vi "Autonomous Independent.vi"   [LabVIEW 2017]
doc: "This VI is called when autonomous begins, and will automatically be terminated when autonomous ends. You can carry out timed or sensor driven robot movement independently without needing to return to the caller."
uses:
  <vilib>/Rock Robotics/Network Tables/NT Read String.vi
  <vilib>/Rock Robotics/WPI/Utilities/WPI_GetSetVariantRefNum.vi
panel:
  # "Be sure to right-click and choose Data Operations>>Make Current Value default if you want to save the array values with the VI"
types:
  T1 = typedef "WPI_GyroDevRef.ctl" = cluster{"DevStatus":errorcluster, "Analog Channel":T2, "Gain (VoltsPerDegree/Second)":dbl, "Gyro Type":enum16{"Analog", "XRS450"}, "Handle":i32, "SPI Bus":T3, "Device Found":bool, "Sample Rate":dbl, "Calibrate On Open":bool, "Offset":dbl}
  T2 = typedef "FPGA_AIChannel.ctl" = enum8{"AI 0", "AI 1", "AI 2", "AI 3", "AI MXP 0", "AI MXP 1", "AI MXP 2", "AI MXP 3", "Invalid"}
  T3 = typedef "spi_bus.ctl" = enum16{"SPI On-Board, CS0", "SPI On-Board, CS1", "SPI On-Board, CS2", "SPI On-Board, CS3", "SPI MXP", "Invalid"}
  T4 = typedef "WPI_EncoderDevRef.ctl" = cluster{"DevStatus":errorcluster, "EncoderIndex":T5, "CounterIndex":T6, "DistancePerCount":dbl, "Decoding Type":T7}
  T5 = typedef "FPGA_EncoderIdx.ctl" = enum8{"Enc 0", "Enc 1", "Enc 2", "Enc 3", "Enc 4", "Enc 5", "Enc 6", "Enc 7", "Invalid"}
  T6 = typedef "FPGA_CounterCtrSystemIndex.ctl" = enum8{"Ctr 0", "Ctr 1", "Ctr 2", "Ctr 3", "Ctr 4", "Ctr 5", "Ctr 6", "Ctr 7", "Invalid"}
  T7 = typedef "WPI_EncoderType.ctl" = enum16{"1x", "2x", "4x"}
  T8 = typedef "WPI_RobotDriveDevRef.ctl" = cluster{"DevStatus":errorcluster, "Motors[]":T9[], "Square Inputs":bool, "Max Output":dbl}
  T9 = typedef "WPI_MotorControlDeviceRef.ctl" = cluster{"DeviceStatus":errorcluster, "Type":T10, "PWM":cluster{"PWM Channel":T11, "DeadBand":T12}, "CAN":cluster{"Device Number":u8, "SetOutput VI Ref":variant, "GetOutput VI Ref":variant, "Enable VI Ref":variant, "Disable VI Ref":variant, "Data":variant}, "Invert":bool, "DIO PWM":cluster{"PWM \"Enable\" Channel":T11, "DIOChannel":T13, "PWM Rate":dbl}}
  T10 = typedef "WPI_MotorControlType.ctl" = enum16{"PWM", "CAN", "DIO PWM"}
  T11 = typedef "FPGA_DIOPWMChannel.ctl" = enum8{"PWM 0", "PWM 1", "PWM 2", "PWM 3", "PWM 4", "PWM 5", "PWM 6", "PWM 7", "PWM 8", "PWM 9", "PWM MXP 0", "PWM MXP 1", "PWM MXP 2", "PWM MXP 3", "PWM MXP 4", "PWM MXP 5", "PWM MXP 6", "PWM MXP 7", "PWM MXP 8", "PWM MXP 9", "Invalid"}
  T12 = typedef "WPI_PWMDeadband.ctl" = cluster{"Name":string, "maxPositivePwm":i32, "minPositivePwm":i32, "centerPwm":i32, "maxNegativePwm":i32, "minNegativePwm":i32, "angularRange":u16}
  T13 = typedef "FPGA_DIOChannel.ctl" = enum8{"DIO 0", "DIO 1", "DIO 2", "DIO 3", "DIO 4", "DIO 5", "DIO 6", "DIO 7", "DIO 8", "DIO 9", "DIO MXP 0", "DIO MXP 1", "DIO MXP 2", "DIO MXP 3", "DIO MXP 4", "DIO MXP 5", "DIO MXP 6", "DIO MXP 7", "DIO MXP 8", "DIO MXP 9", "DIO MXP 10", "DIO MXP 11", "DIO MXP 12", "DIO MXP 13", "DIO MXP 14", "DIO MXP 15", "SPI Port CS1", "SPI Port CS2", "SPI Port CS3", "SPI Port MISO", "SPI Port MOSI", "Invalid"}
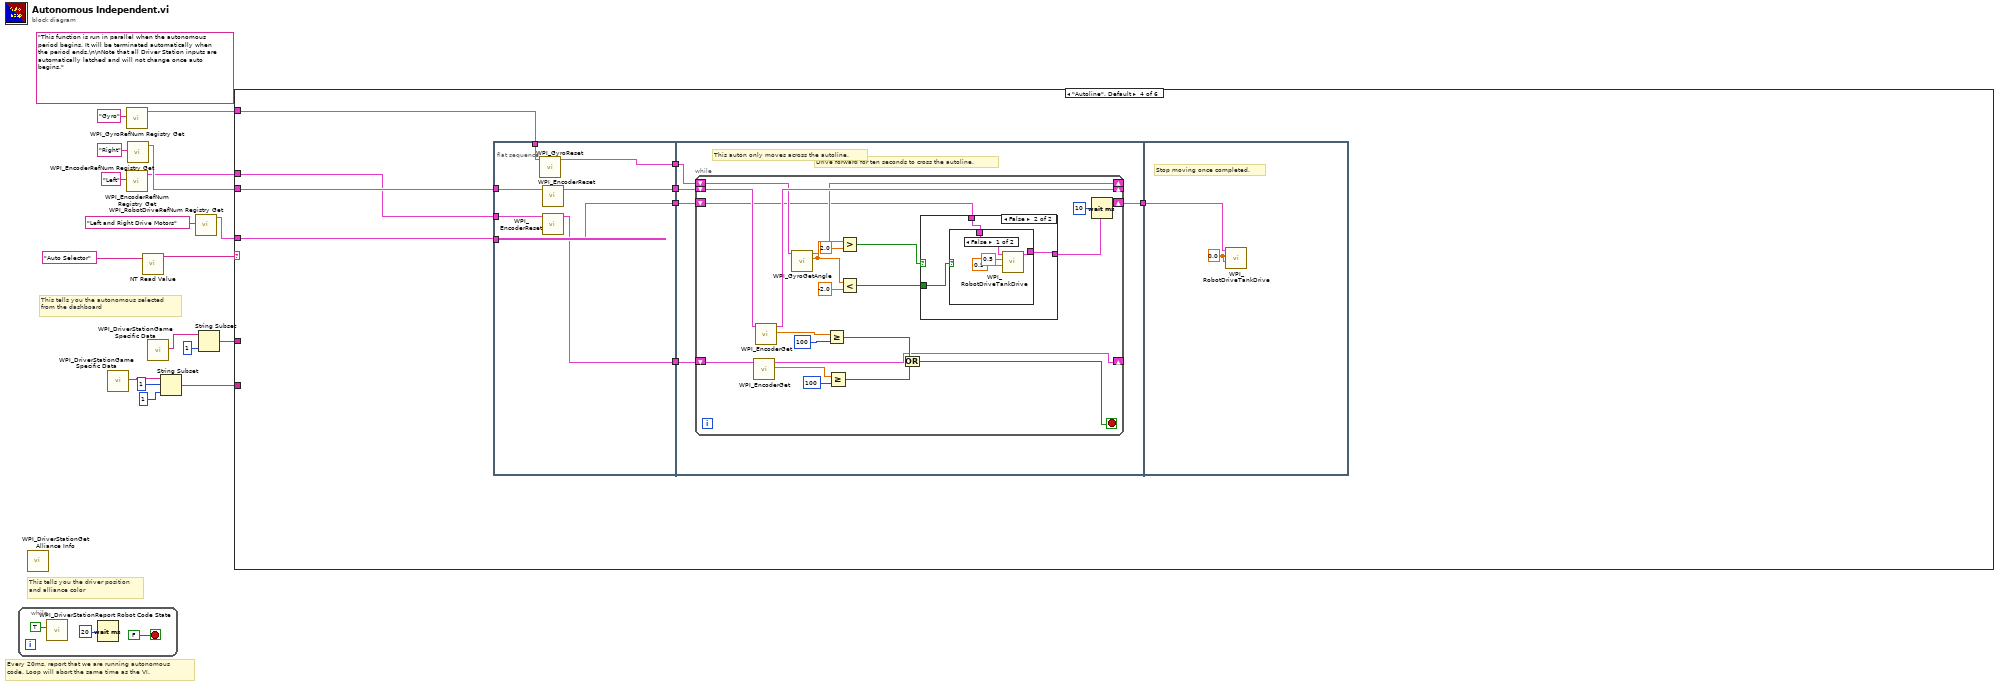
[diagram p0: block diagram]
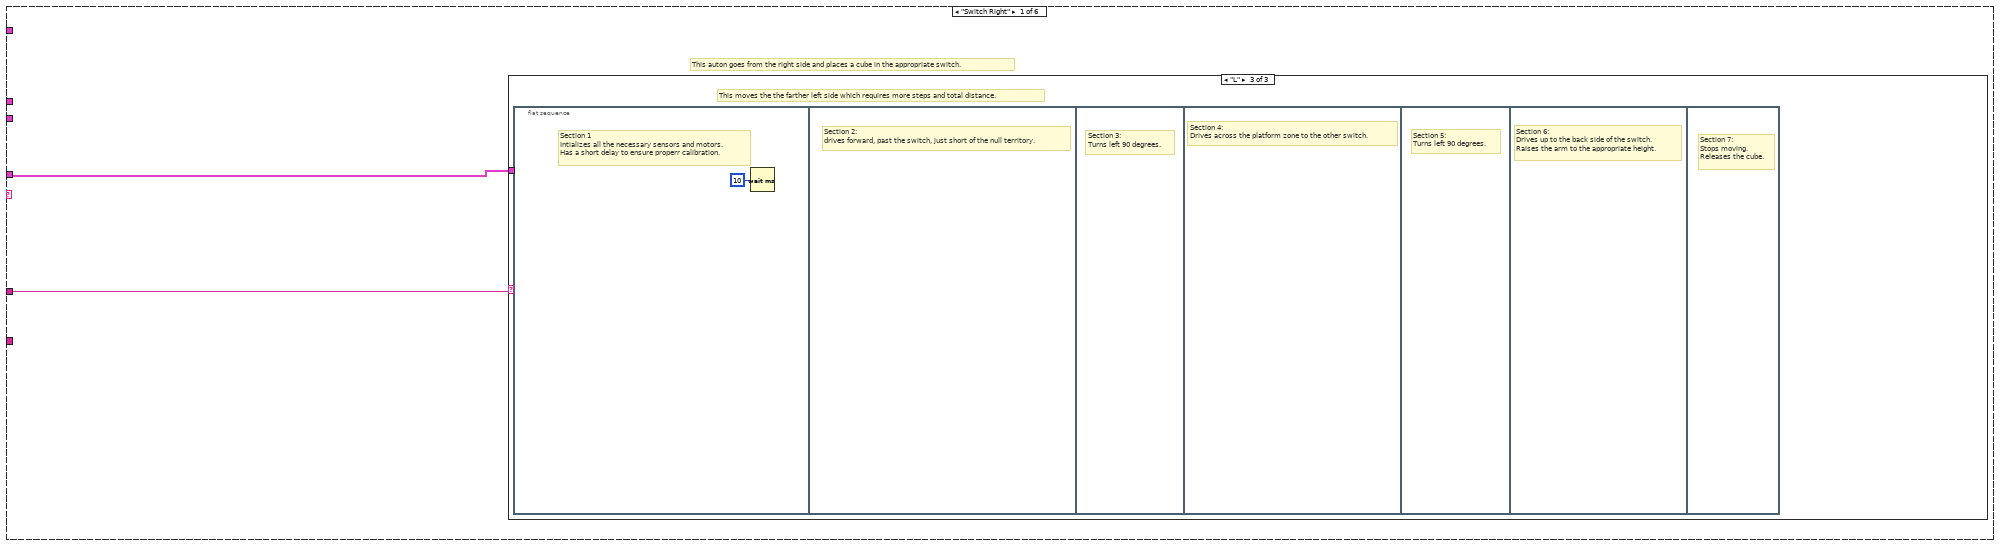
[diagram p2: hidden frame]
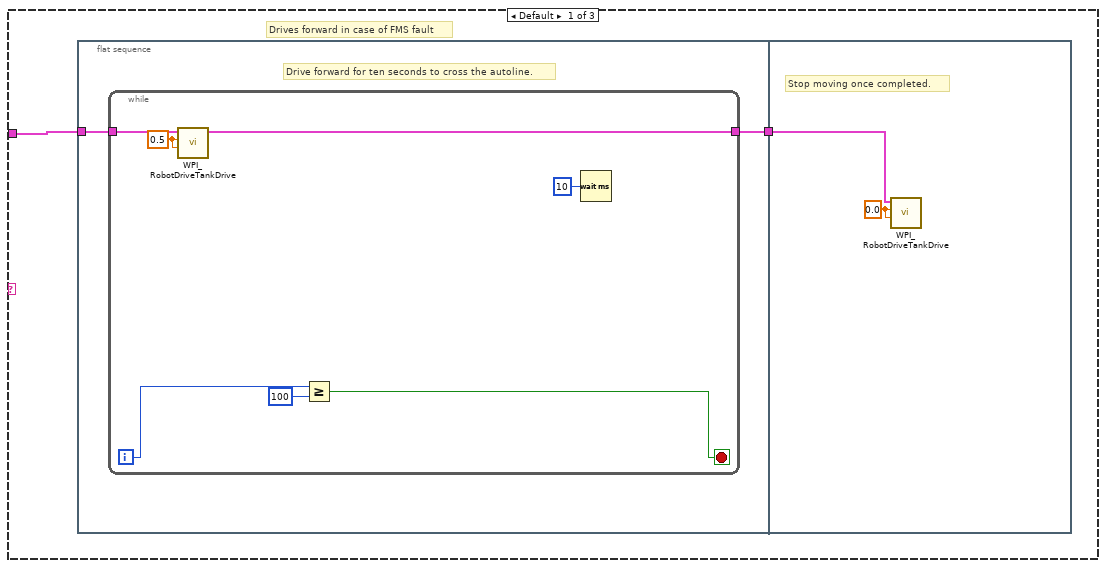
[diagram p3: hidden frame]
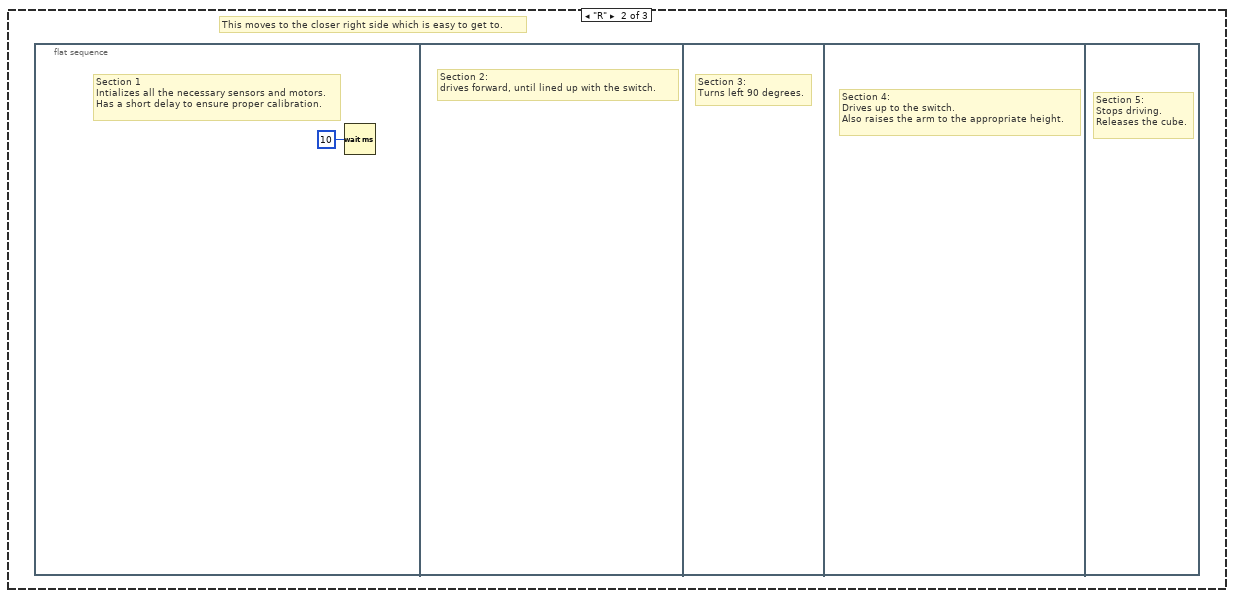
[diagram p4: hidden frame]
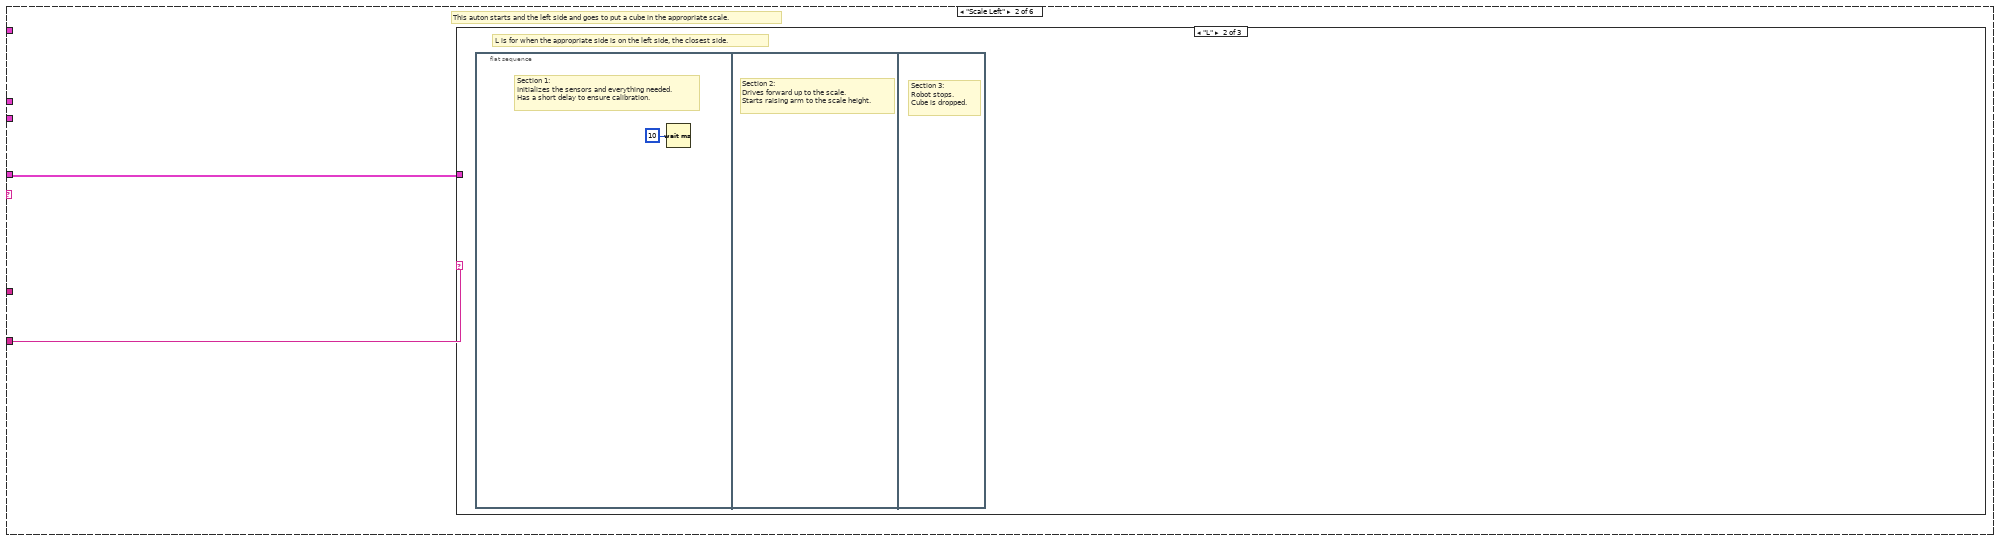
[diagram p5: hidden frame]
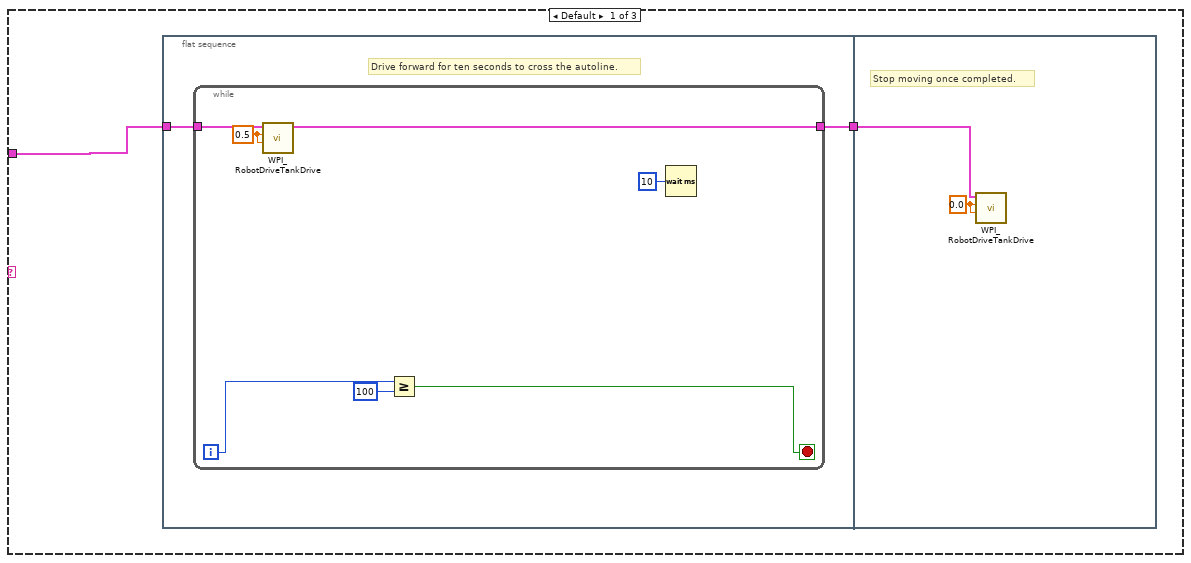
[diagram p6: hidden frame]
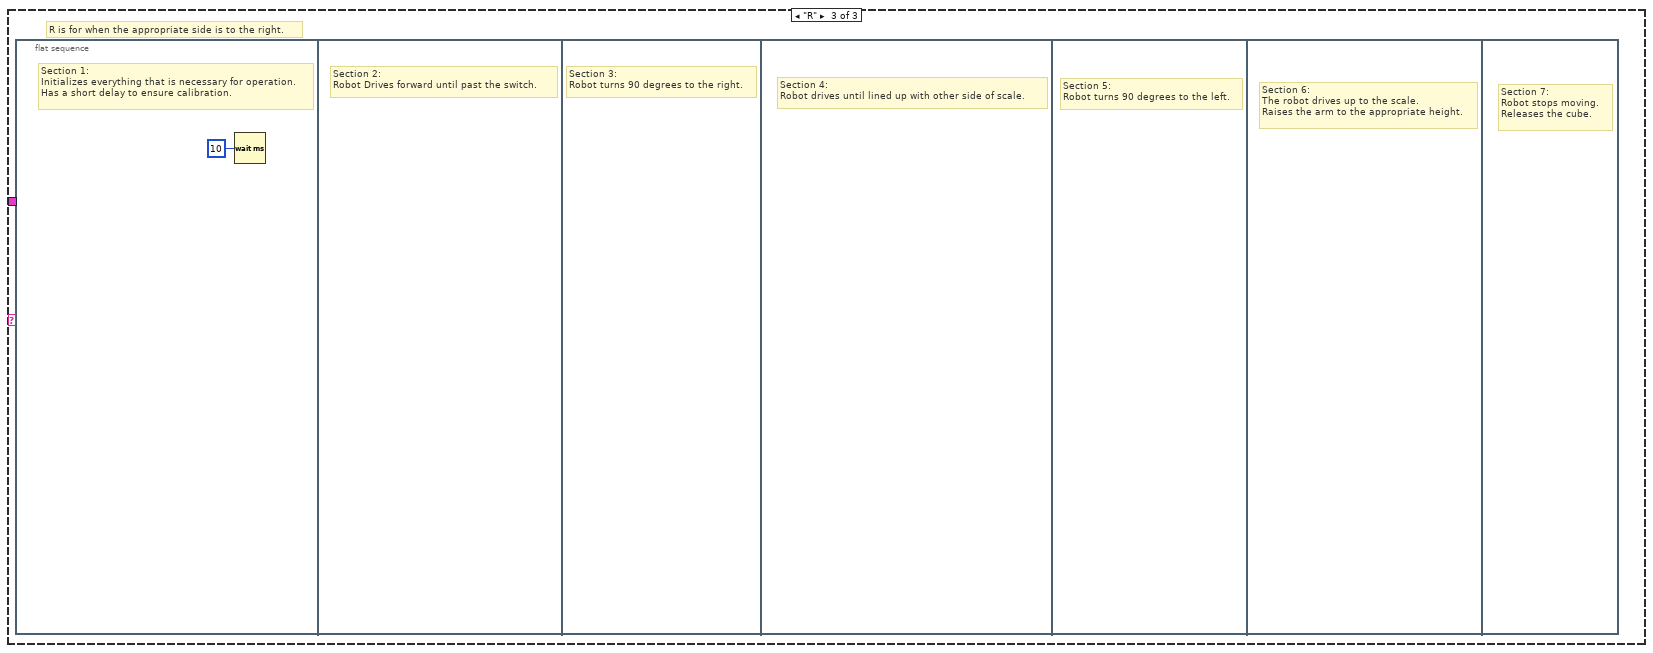
[diagram p7: hidden frame]
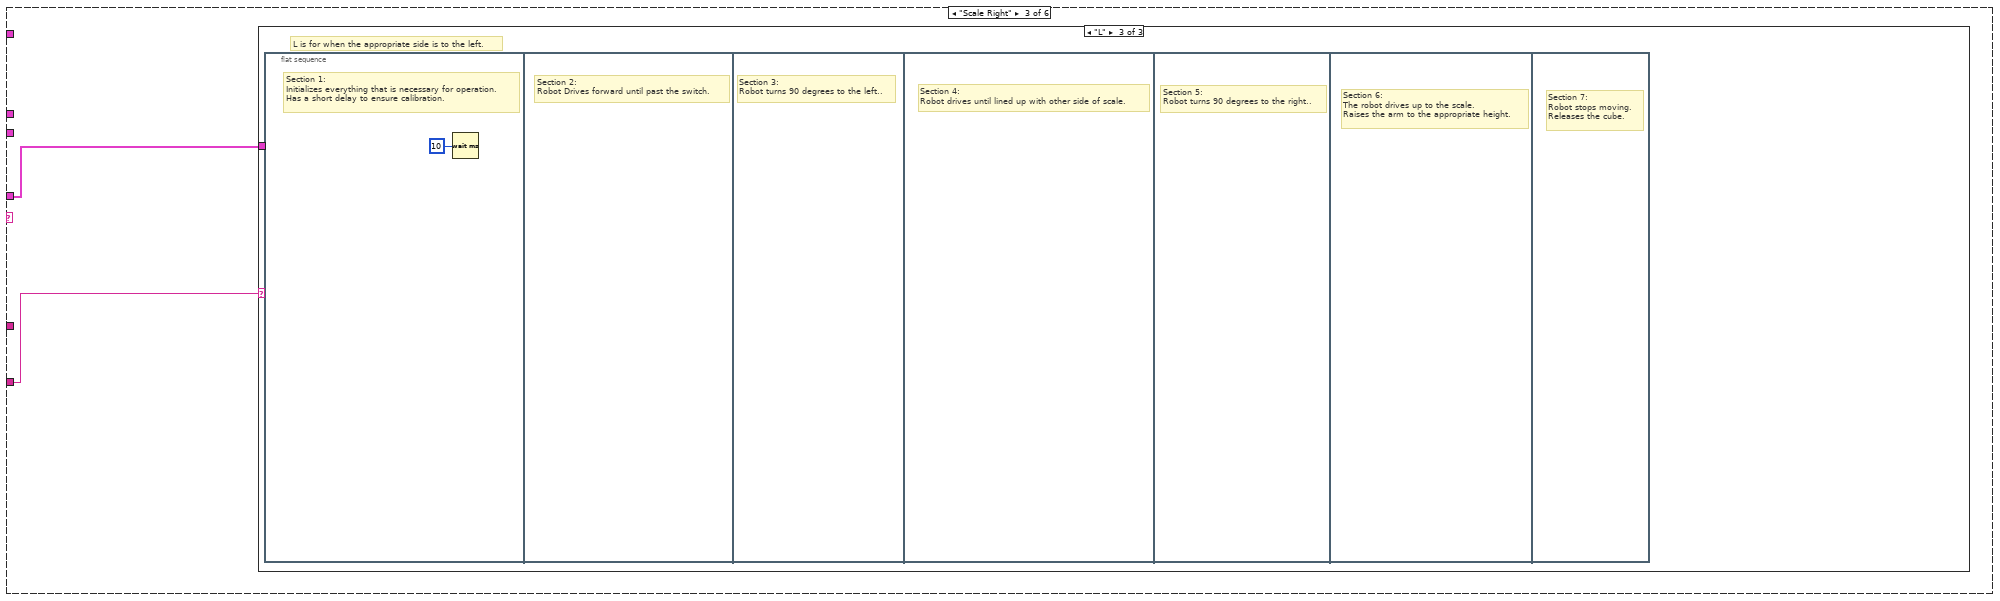
[diagram p8: hidden frame]
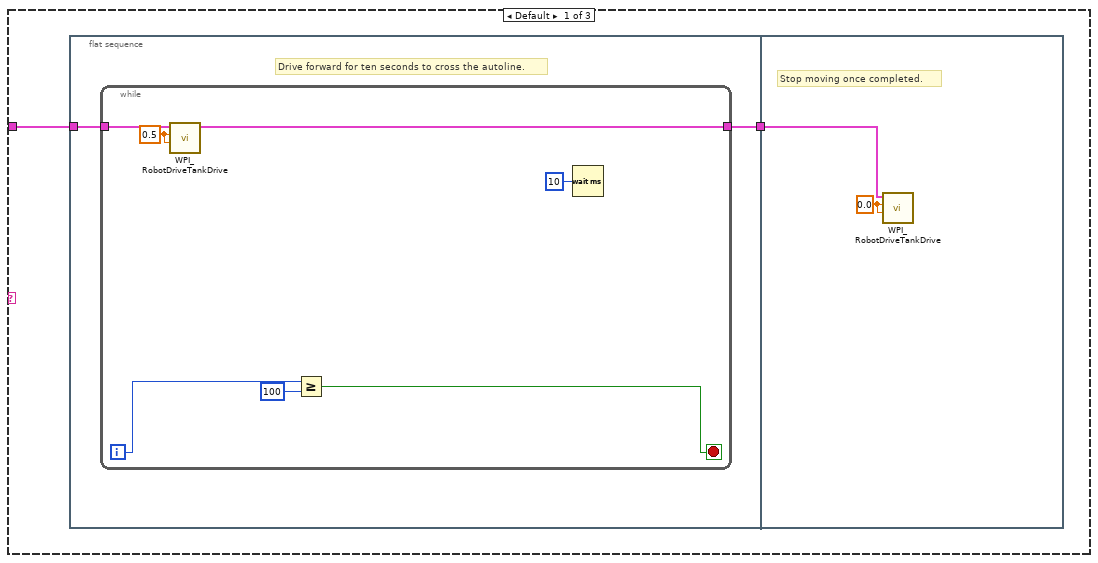
[diagram p9: hidden frame]
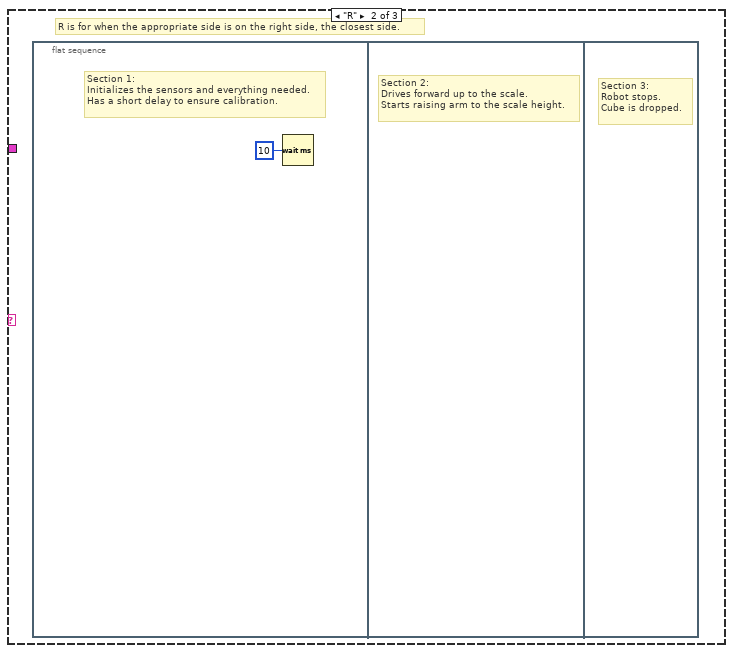
[diagram p10: hidden frame]
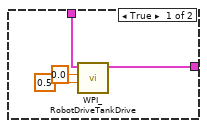
[diagram p11: hidden frame]
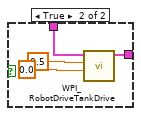
[diagram p12: hidden frame]
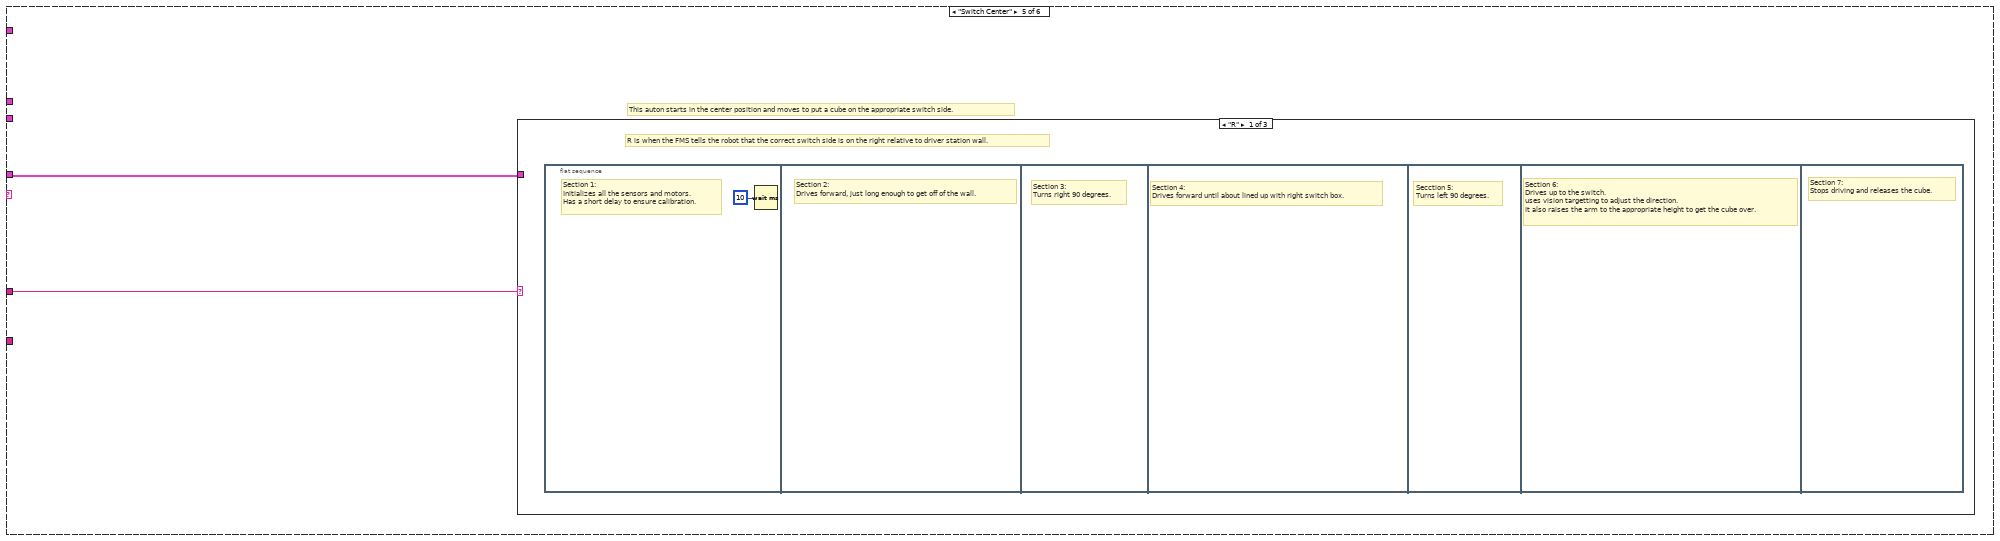
[diagram p13: hidden frame]
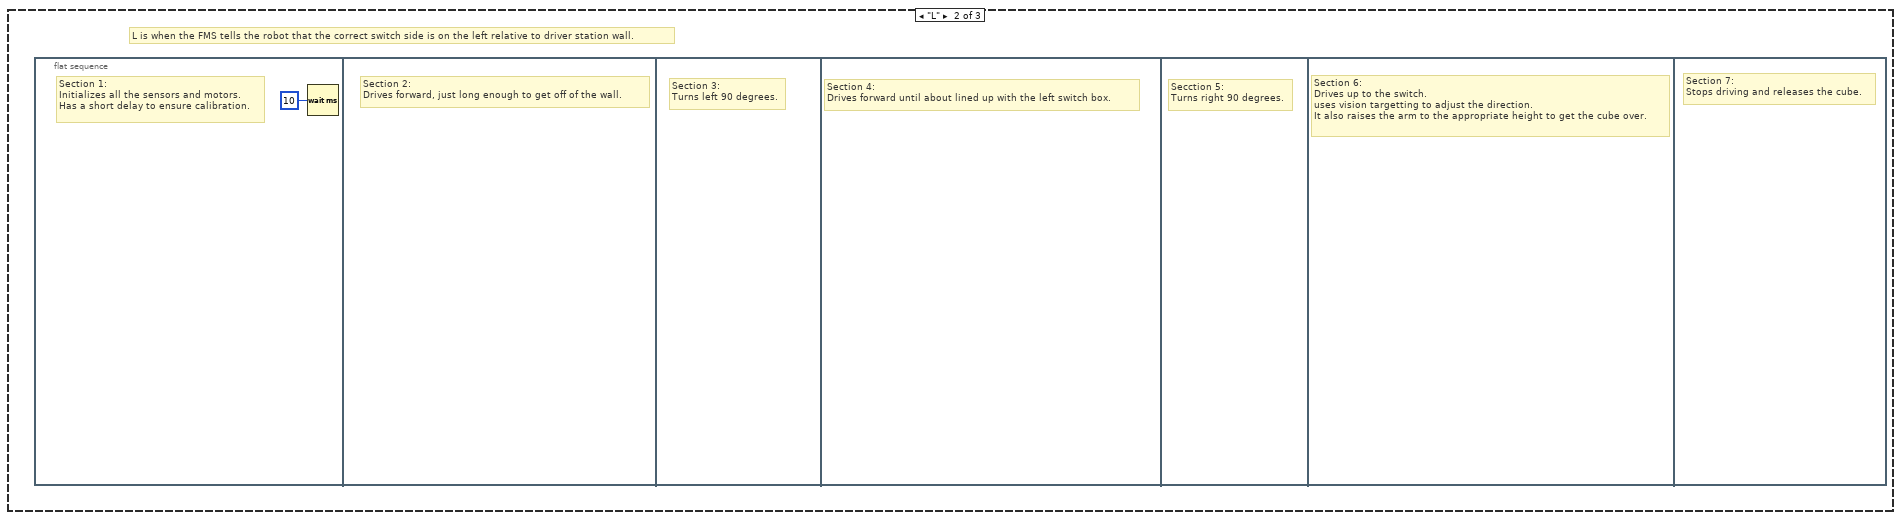
[diagram p14: hidden frame]
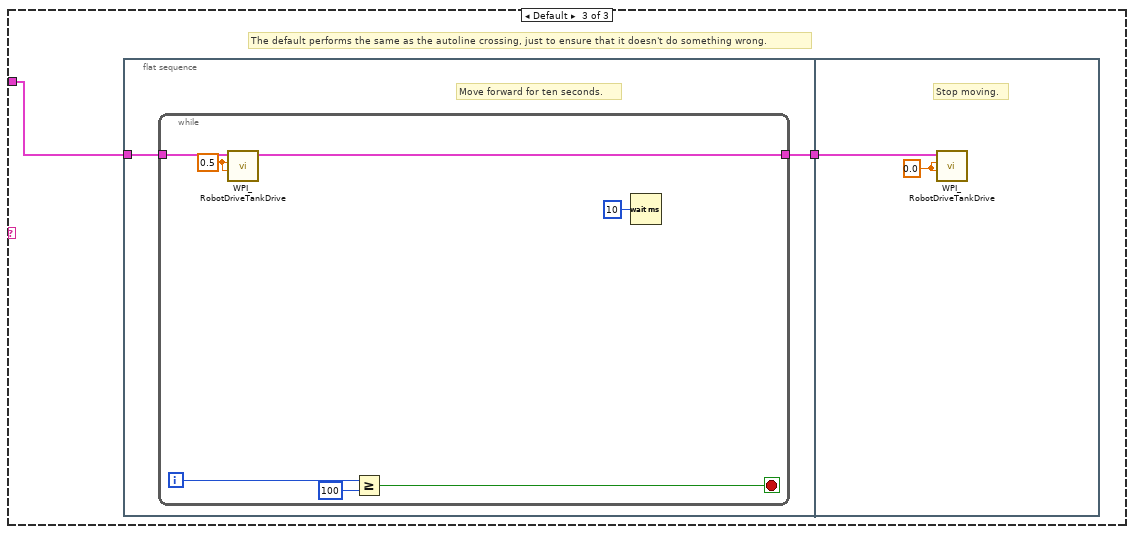
[diagram p15: hidden frame]
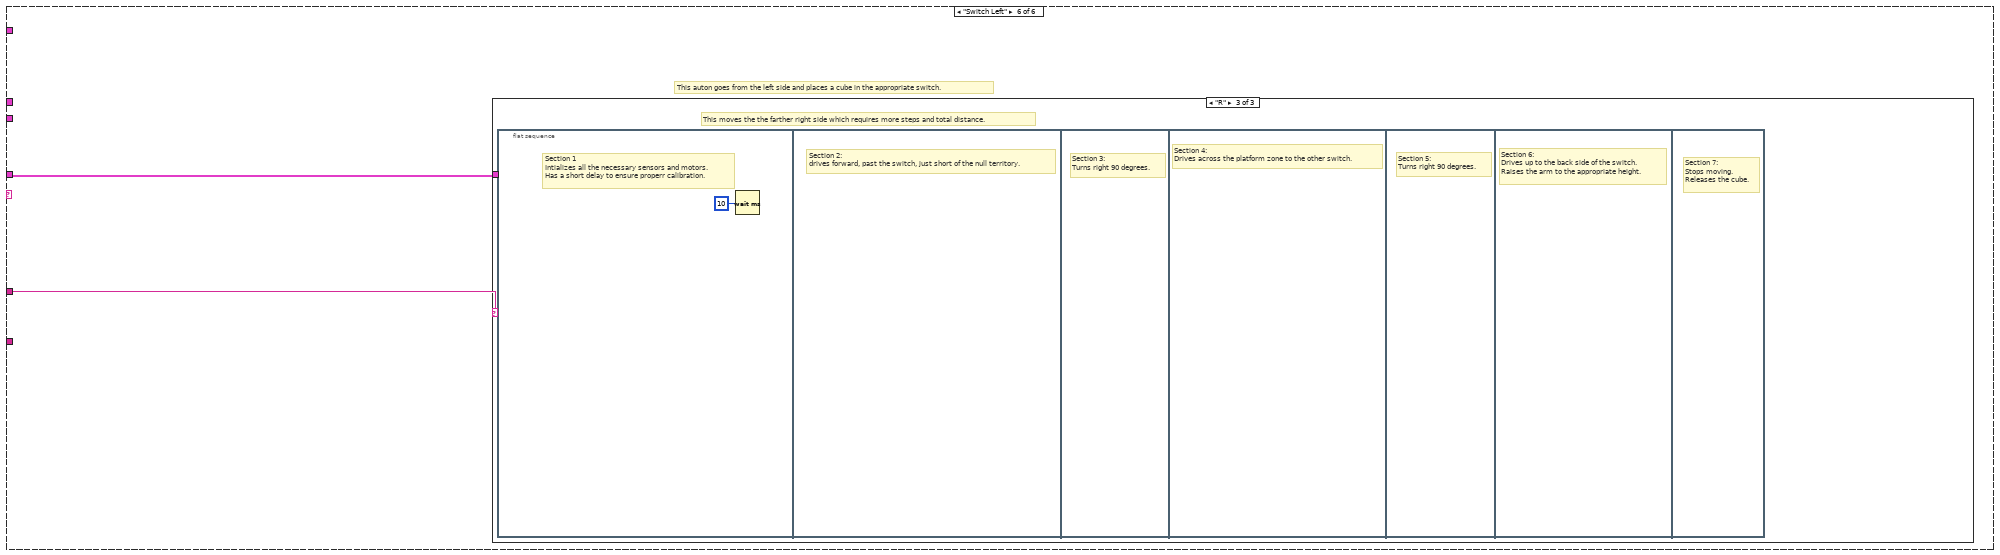
[diagram p16: hidden frame]
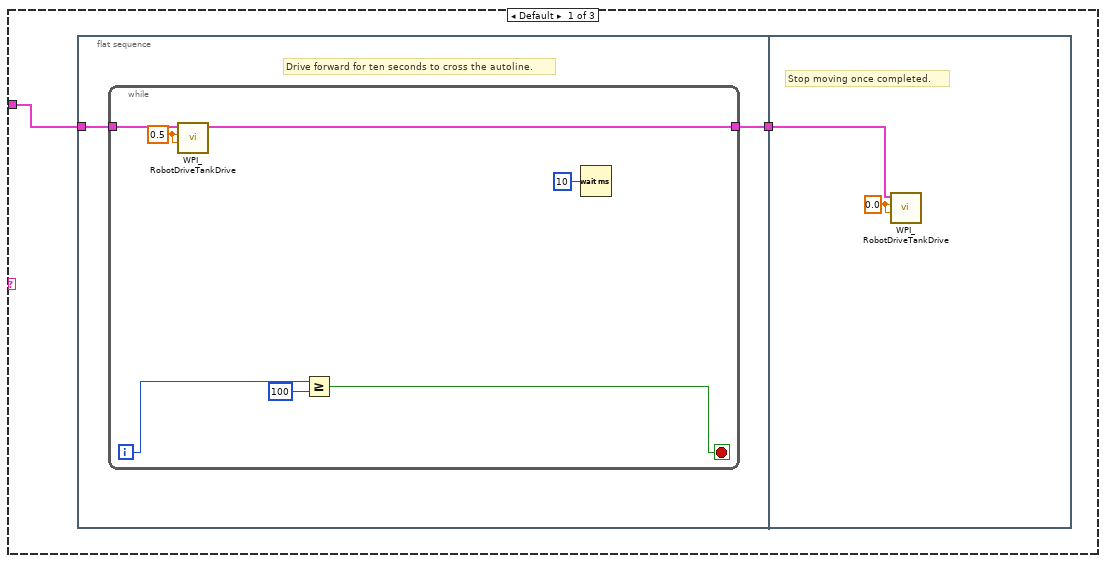
[diagram p17: hidden frame]
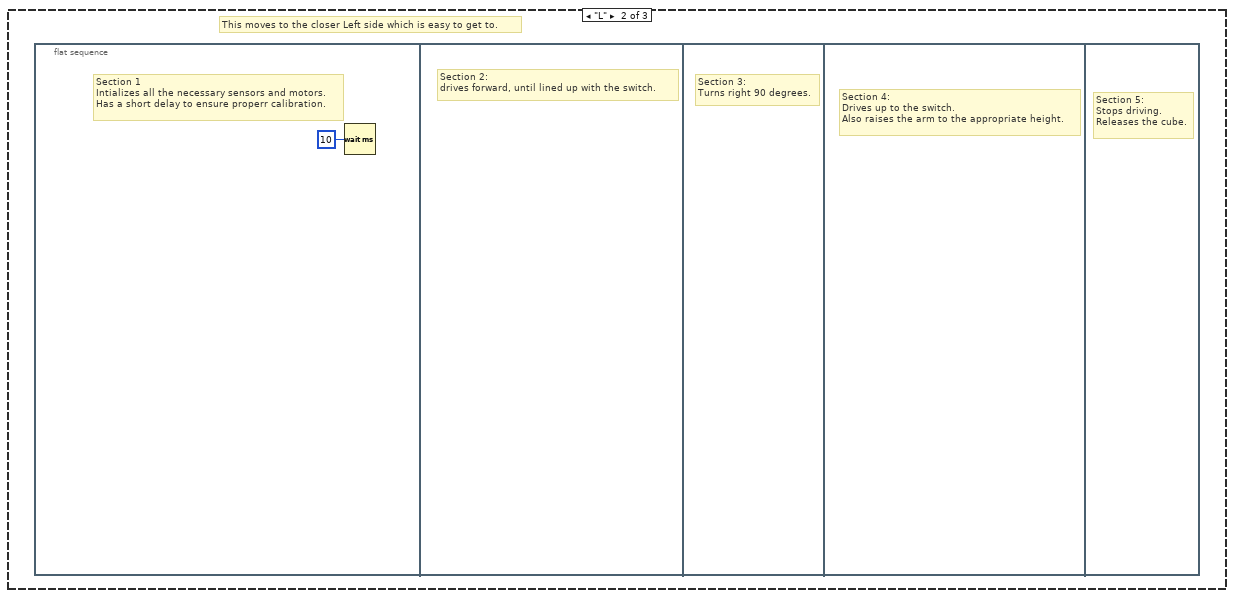
[diagram p18: hidden frame]
diagram:
  (unwired) "This function is run in parallel when the autonomous period begins. It will be terminated automatically when the period ends.\n\nNote that all Driver Station inputs are automatically latched and will not change once auto begins."
  # "This tells you the autonomous selected\nfrom the dashboard"
  # "Every 20ms, report that we are running autonomous\ncode. Loop will abort the same time as the VI."
  # "This tells you the driver position\nand alliance color"
  n1 = while {
    stop <- FALSE stop-if-true
    n2 = call <vilib>:"WPI_DriverStationReport Robot Code State.vi"("Autonomous"=TRUE) -> ()  [unwired: 10 in, 1 out]
    n3 = Wait (ms)(milliseconds to wait=u32 20) -> ()  [unwired: 1 out]
  }
  n4 = call <vilib>:"WPI_DriverStationGet Alliance Info.vi"() -> ()  [unwired: 12 out]
  n5 = call <vilib>:"WPI_DriverStationGame Specific Data.vi"() -> ("Game Specific Data"=w10:string)  [unwired: 11 in]
  n6 = call <vilib>:"WPI_GyroRefNum Registry Get.vi"("refnum name"="Gyro") -> ("GyroDevRef"=w1:T1)  [unwired: 9 in, 1 out]
  n7 = call <vilib>:"WPI_EncoderRefNum Registry Get.vi"("refnum name"="Left") -> ("EncoderDevRef"=w2:T4)  [unwired: 9 in, 1 out]
  n8 = call <vilib>:"WPI_EncoderRefNum Registry Get.vi"("refnum name"="Right") -> ("EncoderDevRef"=w3:T4)  [unwired: 9 in, 1 out]
  n9 = call-poly <vilib>:"NT Read Value.vi"("Name"="Auto Selector") -> ("String"=w16:string)  [unwired: 9 in, 1 out]
  n10 = call <vilib>:"WPI_DriverStationGame Specific Data.vi"() -> ("Game Specific Data"=w13:string)  [unwired: 11 in]
  n11 = String Subset(string=w10, offset (0)=1, length (rest)=1 ("length (rest)")) -> (substring=w7:string)
  n12 = call <vilib>:"WPI_RobotDriveRefNum Registry Get.vi"("refnum name"="Left and Right Drive Motors") -> ("RobotDriveDevRef"=w14:T8)  [unwired: 9 in, 1 out]
  n13 = String Subset(string=w13, length (rest)=1 ("length (rest)")) -> (substring=w11:string)  [unwired: 1 in]
  n14 = case shown="\"Autoline\", Default" w16 {
    tunnel: w14 -> [w22 w38 w55 w80 w131 w148]
    tunnel: w11 -> [w21 _ _ _ w132 w149]
    tunnel: w7 -> [_ w39 w56 _ _ _]
    tunnel: w3 -> [_ _ _ w78 _ _]
    tunnel: w2 -> [_ _ _ w76 _ _]
    tunnel: w1 -> [_ _ _ w74 _ _]
    frame "Switch Right" {
      # "This auton goes from the right side and places a cube in the appropriate switch."
      n15 = case shown="\"L\"" w21 {
        tunnel: w22 -> [w23 _ _]
        frame Default {
          # "Drives forward in case of FMS fault"
          n16 = flat-sequence {
            tunnel: w23 -> [w26]
            tunnel: [w25] -> w24
            tunnel: w24 -> [w34]
            frame #0 {
              # "Drive forward for ten seconds to cross the autoline."
              n17 = while {
                tunnel: w26 -> [w33]
                tunnel: [w27] -> w25
                i -> [w31]
                stop <- w28 stop-if-true
                w32 = 0.5 ("Left axis value")
                n18 = call <vilib>:"WPI_RobotDriveTankDrive.vi"("Right axis value"=w32, "Left axis value"=w32, "RobotDriveDevRef"=w33) -> ("RobotDriveDevRef"=w27:T8)  [unwired: 6 in, 2 out]
                n19 = Greater Or Equal?(x=w31, y=100) -> (x >= y?=w28:bool)
                n20 = Wait (ms)(milliseconds to wait=u32 10) -> ()  [unwired: 1 out]
              }
            }
            frame #1 {
              w35 = 0.0 ("Left axis value")
              # "Stop moving once completed."
              n21 = call <vilib>:"WPI_RobotDriveTankDrive.vi"("Right axis value"=w35, "Left axis value"=w35, "RobotDriveDevRef"=w34) -> ()  [unwired: 6 in, 3 out]
            }
          }
        }
        frame "R" {
          # "This moves to the closer right side which is easy to get to."
          n22 = flat-sequence {
            frame #0 {
              # "Section 1\nIntializes all the necessary sensors and motors.\nHas a short delay to ensure proper calibration."
              n23 = Wait (ms)(milliseconds to wait=u32 10) -> ()  [unwired: 1 out]
            }
            frame #1 {
              # "Section 2:\ndrives forward, until lined up with the switch."
            }
            frame #2 {
              # "Section 3:\nTurns left 90 degrees."
            }
            frame #3 {
              # "Section 4:\nDrives up to the switch.\nAlso raises the arm to the appropriate height."
            }
            frame #4 {
              # "Section 5: \nStops driving.\nReleases the cube."
            }
          }
        }
        frame "L" {
          # "This moves the the farther left side which requires more steps and total distance."
          n24 = flat-sequence {
            frame #0 {
              # "Section 1\nIntializes all the necessary sensors and motors.\nHas a short delay to ensure properr calibration."
              n25 = Wait (ms)(milliseconds to wait=u32 10) -> ()  [unwired: 1 out]
            }
            frame #1 {
              # "Section 2:\ndrives forward, past the switch, just short of the null territory."
            }
            frame #2 {
              # "Section 3:\nTurns left 90 degrees."
            }
            frame #3 {
              # "Section 4:\nDrives across the platform zone to the other switch."
            }
            frame #4 {
              # "Section 5:\nTurns left 90 degrees."
            }
            frame #5 {
              # "Section 6:\nDrives up to the back side of the switch.\nRaises the arm to the appropriate height."
            }
            frame #6 {
              # "Section 7:\nStops moving.\nReleases the cube."
            }
          }
        }
      }
    }
    frame "Scale Left" {
      # "This auton starts and the left side and goes to put a cube in the appropriate scale."
      n26 = case shown="\"L\"" w39 {
        tunnel: w38 -> [w40 _ _]
        frame Default {
          n27 = flat-sequence {
            tunnel: w40 -> [w42]
            tunnel: [w43] -> w41
            tunnel: w41 -> [w51]
            frame #0 {
              # "Drive forward for ten seconds to cross the autoline."
              n28 = while {
                tunnel: w42 -> [w50]
                tunnel: [w44] -> w43
                i -> [w48]
                stop <- w45 stop-if-true
                w49 = 0.5 ("Left axis value")
                n29 = call <vilib>:"WPI_RobotDriveTankDrive.vi"("Right axis value"=w49, "Left axis value"=w49, "RobotDriveDevRef"=w50) -> ("RobotDriveDevRef"=w44:T8)  [unwired: 6 in, 2 out]
                n30 = Greater Or Equal?(x=w48, y=100) -> (x >= y?=w45:bool)
                n31 = Wait (ms)(milliseconds to wait=u32 10) -> ()  [unwired: 1 out]
              }
            }
            frame #1 {
              w52 = 0.0 ("Left axis value")
              # "Stop moving once completed."
              n32 = call <vilib>:"WPI_RobotDriveTankDrive.vi"("Right axis value"=w52, "Left axis value"=w52, "RobotDriveDevRef"=w51) -> ()  [unwired: 6 in, 3 out]
            }
          }
        }
        frame "L" {
          # "L is for when the appropriate side is on the left side, the closest side."
          n33 = flat-sequence {
            frame #0 {
              # "Section 1:\nInitializes the sensors and everything needed.\nHas a short delay to ensure calibration."
              n34 = Wait (ms)(milliseconds to wait=u32 10) -> ()  [unwired: 1 out]
            }
            frame #1 {
              # "Section 2:\nDrives forward up to the scale.\nStarts raising arm to the scale height."
            }
            frame #2 {
              # "Section 3:\nRobot stops.\nCube is dropped."
            }
          }
        }
        frame "R" {
          # "R is for when the appropriate side is to the right."
          n35 = flat-sequence {
            frame #0 {
              # "Section 1:\nInitializes everything that is necessary for operation.\nHas a short delay to ensure calibration."
              n36 = Wait (ms)(milliseconds to wait=u32 10) -> ()  [unwired: 1 out]
            }
            frame #1 {
              # "Section 2:\nRobot Drives forward until past the switch."
            }
            frame #2 {
              # "Section 3:\nRobot turns 90 degrees to the right."
            }
            frame #3 {
              # "Section 4:\nRobot drives until lined up with other side of scale."
            }
            frame #4 {
              # "Section 5:\nRobot turns 90 degrees to the left."
            }
            frame #5 {
              # "Section 6:\nThe robot drives up to the scale.\nRaises the arm to the appropriate height."
            }
            frame #6 {
              # "Section 7:\nRobot stops moving.\nReleases the cube."
            }
          }
        }
      }
    }
    frame "Scale Right" {
      n37 = case shown="\"L\"" w56 {
        tunnel: w55 -> [w57 _ _]
        frame Default {
          n38 = flat-sequence {
            tunnel: w57 -> [w60]
            tunnel: [w59] -> w58
            tunnel: w58 -> [w68]
            frame #0 {
              # "Drive forward for ten seconds to cross the autoline."
              n39 = while {
                tunnel: w60 -> [w67]
                tunnel: [w61] -> w59
                i -> [w65]
                stop <- w62 stop-if-true
                w66 = 0.5 ("Left axis value")
                n40 = call <vilib>:"WPI_RobotDriveTankDrive.vi"("Right axis value"=w66, "Left axis value"=w66, "RobotDriveDevRef"=w67) -> ("RobotDriveDevRef"=w61:T8)  [unwired: 6 in, 2 out]
                n41 = Greater Or Equal?(x=w65, y=100) -> (x >= y?=w62:bool)
                n42 = Wait (ms)(milliseconds to wait=u32 10) -> ()  [unwired: 1 out]
              }
            }
            frame #1 {
              w69 = 0.0 ("Left axis value")
              # "Stop moving once completed."
              n43 = call <vilib>:"WPI_RobotDriveTankDrive.vi"("Right axis value"=w69, "Left axis value"=w69, "RobotDriveDevRef"=w68) -> ()  [unwired: 6 in, 3 out]
            }
          }
        }
        frame "R" {
          # "R is for when the appropriate side is on the right side, the closest side."
          n44 = flat-sequence {
            frame #0 {
              # "Section 1:\nInitializes the sensors and everything needed.\nHas a short delay to ensure calibration."
              n45 = Wait (ms)(milliseconds to wait=u32 10) -> ()  [unwired: 1 out]
            }
            frame #1 {
              # "Section 2:\nDrives forward up to the scale.\nStarts raising arm to the scale height."
            }
            frame #2 {
              # "Section 3:\nRobot stops.\nCube is dropped."
            }
          }
        }
        frame "L" {
          # "L is for when the appropriate side is to the left."
          n46 = flat-sequence {
            frame #0 {
              # "Section 1:\nInitializes everything that is necessary for operation.\nHas a short delay to ensure calibration."
              n47 = Wait (ms)(milliseconds to wait=u32 10) -> ()  [unwired: 1 out]
            }
            frame #1 {
              # "Section 2:\nRobot Drives forward until past the switch."
            }
            frame #2 {
              # "Section 3:\nRobot turns 90 degrees to the left.."
            }
            frame #3 {
              # "Section 4:\nRobot drives until lined up with other side of scale."
            }
            frame #4 {
              # "Section 5:\nRobot turns 90 degrees to the right.."
            }
            frame #5 {
              # "Section 6:\nThe robot drives up to the scale.\nRaises the arm to the appropriate height."
            }
            frame #6 {
              # "Section 7:\nRobot stops moving.\nReleases the cube."
            }
          }
        }
      }
    }
    frame "Autoline", Default {
      n48 = flat-sequence {
        tunnel: w80 -> [w87]
        tunnel: [w87] -> w79
        tunnel: w78 -> [w86]
        tunnel: [w85] -> w77
        tunnel: w76 -> [w84]
        tunnel: [w83] -> w75
        tunnel: w74 -> [w82]
        tunnel: [w81] -> w73
        tunnel: w79 -> [w92]
        tunnel: w77 -> [w91]
        tunnel: w75 -> [w90]
        tunnel: w73 -> [w89]
        tunnel: [w88] -> w72
        tunnel: w72 -> [w129]
        frame #0 {
          n49 = call <vilib>:"WPI_GyroReset.vi"("GyroDevRef"=w82) -> ("GyroDevRef"=w81:T1)  [unwired: 9 in, 1 out]
          n50 = call <vilib>:"WPI_EncoderReset.vi"("EncoderDevRef"=w86) -> ("EncoderDevRef"=w85:T4)  [unwired: 9 in, 1 out]
          n51 = call <vilib>:"WPI_EncoderReset.vi"("EncoderDevRef"=w84) -> ("EncoderDevRef"=w83:T4)  [unwired: 9 in, 1 out]
        }
        frame #1 {
          # "This auton only moves across the autoline."
          # "Drive forward for ten seconds to cross the autoline."
          n52 = while {
            shift-right: [w102] -> _
            shift-left: w90 -> [w104]
            shift-right: [w103] -> _
            shift-left: w91 -> [w105]
            shift-right: [w99] -> _
            shift-left: w89 -> [w100]
            shift-right: [w94] -> w88
            shift-left: w92 -> [w95]
            stop <- w108 stop-if-true
            n53 = call <vilib>:"WPI_EncoderGet.vi"("EncoderDevRef"=w104) -> ("Distance"=w107:dbl, "EncoderDevRef"=w102:T4)  [unwired: 5 in, 4 out]
            n54 = call <vilib>:"WPI_EncoderGet.vi"("EncoderDevRef"=w105) -> ("Distance"=w106:dbl, "EncoderDevRef"=w103:T4)  [unwired: 5 in, 4 out]
            n55 = call <vilib>:"WPI_GyroGetAngle.vi"("GyroDevRef"=w100) -> ("Angle"=w101:dbl, "GyroDevRef"=w99:T1)  [unwired: 6 in, 3 out]
            n56 = Greater Or Equal?(x=w106, y=100) -> (x >= y?=w110:bool)
            n57 = Greater Or Equal?(x=w107, y=100) -> (x >= y?=w109:bool)
            n58 = Greater?(x=w101, y=2.0) -> (0:w96:bool)
            n59 = Less?(x=w101, y=-2.0) -> (x < y?=w93:bool)
            n60 = Or(x=w110, y=w109) -> (x .or. y?=w108:bool)
            n61 = case shown="False" w96 {
              tunnel: w95 -> [w115 w119]
              tunnel: [w114 w118] -> w94
              tunnel: w93 -> [_ w120]
              frame True {
                n62 = call <vilib>:"WPI_RobotDriveTankDrive.vi"("Right axis value"=0.5, "Left axis value"=0.0, "RobotDriveDevRef"=w115) -> ("RobotDriveDevRef"=w114:T8)  [unwired: 6 in, 2 out]
              }
              frame False {
                n63 = case shown="False" w120 {
                  tunnel: w119 -> [w122 w126]
                  tunnel: [w121 w125] -> w118
                  frame False {
                    n64 = call <vilib>:"WPI_RobotDriveTankDrive.vi"("Right axis value"=0.5, "Left axis value"=0.5, "RobotDriveDevRef"=w122) -> ("RobotDriveDevRef"=w121:T8)  [unwired: 6 in, 2 out]
                  }
                  frame True {
                    n65 = call <vilib>:"WPI_RobotDriveTankDrive.vi"("Right axis value"=0.0, "Left axis value"=0.5, "RobotDriveDevRef"=w126) -> ("RobotDriveDevRef"=w125:T8)  [unwired: 6 in, 2 out]
                  }
                }
              }
            }
            n66 = Wait (ms)(milliseconds to wait=u32 10) -> ()  [unwired: 1 out]
          }
        }
        frame #2 {
          w130 = 0.0 ("Left axis value")
          # "Stop moving once completed."
          n67 = call <vilib>:"WPI_RobotDriveTankDrive.vi"("Right axis value"=w130, "Left axis value"=w130, "RobotDriveDevRef"=w129) -> ()  [unwired: 6 in, 3 out]
        }
      }
    }
    frame "Switch Center" {
      # "This auton starts in the center position and moves to put a cube on the appropriate switch side."
      n68 = case shown="\"R\"" w132 {
        tunnel: w131 -> [_ _ w135]
        frame "R" {
          # "R is when the FMS tells the robot that the correct switch side is on the right relative to driver station wall."
          n69 = flat-sequence {
            frame #0 {
              # "Section 1:\nInitializes all the sensors and motors.\nHas a short delay to ensure calibration."
              n70 = Wait (ms)(milliseconds to wait=u32 10) -> ()  [unwired: 1 out]
            }
            frame #1 {
              # "Section 2:\nDrives forward, just long enough to get off of the wall."
            }
            frame #2 {
              # "Section 3:\nTurns right 90 degrees."
            }
            frame #3 {
              # "Section 4:\nDrives forward until about lined up with right switch box."
            }
            frame #4 {
              # "Secction 5:\nTurns left 90 degrees."
            }
            frame #5 {
              # "Section 6:\nDrives up to the switch.\nuses vision targetting to adjust the direction.\nIt also raises the arm to the appropriate height to get the cube over."
            }
            frame #6 {
              # "Section 7:\nStops driving and releases the cube."
            }
          }
        }
        frame "L" {
          # "L is when the FMS tells the robot that the correct switch side is on the left relative to driver station wall."
          n71 = flat-sequence {
            frame #0 {
              # "Section 1:\nInitializes all the sensors and motors.\nHas a short delay to ensure calibration."
              n72 = Wait (ms)(milliseconds to wait=u32 10) -> ()  [unwired: 1 out]
            }
            frame #1 {
              # "Section 2:\nDrives forward, just long enough to get off of the wall."
            }
            frame #2 {
              # "Section 3:\nTurns left 90 degrees."
            }
            frame #3 {
              # "Section 4:\nDrives forward until about lined up with the left switch box."
            }
            frame #4 {
              # "Secction 5:\nTurns right 90 degrees."
            }
            frame #5 {
              # "Section 6:\nDrives up to the switch.\nuses vision targetting to adjust the direction.\nIt also raises the arm to the appropriate height to get the cube over."
            }
            frame #6 {
              # "Section 7:\nStops driving and releases the cube."
            }
          }
        }
        frame Default {
          # "The default performs the same as the autoline crossing, just to ensure that it doesn't do something wrong."
          n73 = flat-sequence {
            tunnel: w135 -> [w138]
            tunnel: [w137] -> w136
            tunnel: w136 -> [w146]
            frame #0 {
              # "Move forward for ten seconds."
              n74 = while {
                tunnel: w138 -> [w145]
                tunnel: [w139] -> w137
                i -> [w143]
                stop <- w140 stop-if-true
                w144 = 0.5 ("Left axis value")
                n75 = call <vilib>:"WPI_RobotDriveTankDrive.vi"("Right axis value"=w144, "Left axis value"=w144, "RobotDriveDevRef"=w145) -> ("RobotDriveDevRef"=w139:T8)  [unwired: 6 in, 2 out]
                n76 = Greater Or Equal?(x=w143, y=100) -> (x >= y?=w140:bool)
                n77 = Wait (ms)(milliseconds to wait=u32 10) -> ()  [unwired: 1 out]
              }
            }
            frame #1 {
              w147 = 0.0 ("Left axis value")
              # "Stop moving."
              n78 = call <vilib>:"WPI_RobotDriveTankDrive.vi"("Right axis value"=w147, "Left axis value"=w147, "RobotDriveDevRef"=w146) -> ()  [unwired: 6 in, 3 out]
            }
          }
        }
      }
    }
    frame "Switch Left" {
      # "This auton goes from the left side and places a cube in the appropriate switch."
      n79 = case shown="\"R\"" w149 {
        tunnel: w148 -> [w150 _ _]
        frame Default {
          n80 = flat-sequence {
            tunnel: w150 -> [w153]
            tunnel: [w152] -> w151
            tunnel: w151 -> [w161]
            frame #0 {
              # "Drive forward for ten seconds to cross the autoline."
              n81 = while {
                tunnel: w153 -> [w160]
                tunnel: [w154] -> w152
                i -> [w158]
                stop <- w155 stop-if-true
                w159 = 0.5 ("Left axis value")
                n82 = call <vilib>:"WPI_RobotDriveTankDrive.vi"("Right axis value"=w159, "Left axis value"=w159, "RobotDriveDevRef"=w160) -> ("RobotDriveDevRef"=w154:T8)  [unwired: 6 in, 2 out]
                n83 = Greater Or Equal?(x=w158, y=100) -> (x >= y?=w155:bool)
                n84 = Wait (ms)(milliseconds to wait=u32 10) -> ()  [unwired: 1 out]
              }
            }
            frame #1 {
              w162 = 0.0 ("Left axis value")
              # "Stop moving once completed."
              n85 = call <vilib>:"WPI_RobotDriveTankDrive.vi"("Right axis value"=w162, "Left axis value"=w162, "RobotDriveDevRef"=w161) -> ()  [unwired: 6 in, 3 out]
            }
          }
        }
        frame "L" {
          # "This moves to the closer Left side which is easy to get to."
          n86 = flat-sequence {
            frame #0 {
              # "Section 1\nIntializes all the necessary sensors and motors.\nHas a short delay to ensure properr calibration."
              n87 = Wait (ms)(milliseconds to wait=u32 10) -> ()  [unwired: 1 out]
            }
            frame #1 {
              # "Section 2:\ndrives forward, until lined up with the switch."
            }
            frame #2 {
              # "Section 3:\nTurns right 90 degrees."
            }
            frame #3 {
              # "Section 4:\nDrives up to the switch.\nAlso raises the arm to the appropriate height."
            }
            frame #4 {
              # "Section 5: \nStops driving.\nReleases the cube."
            }
          }
        }
        frame "R" {
          # "This moves the the farther right side which requires more steps and total distance."
          n88 = flat-sequence {
            frame #0 {
              # "Section 1\nIntializes all the necessary sensors and motors.\nHas a short delay to ensure properr calibration."
              n89 = Wait (ms)(milliseconds to wait=u32 10) -> ()  [unwired: 1 out]
            }
            frame #1 {
              # "Section 2:\ndrives forward, past the switch, just short of the null territory."
            }
            frame #2 {
              # "Section 3:\nTurns right 90 degrees."
            }
            frame #3 {
              # "Section 4:\nDrives across the platform zone to the other switch."
            }
            frame #4 {
              # "Section 5:\nTurns right 90 degrees."
            }
            frame #5 {
              # "Section 6:\nDrives up to the back side of the switch.\nRaises the arm to the appropriate height."
            }
            frame #6 {
              # "Section 7:\nStops moving.\nReleases the cube."
            }
          }
        }
      }
    }
  }
